vi "main.vi"() -> ()   [LabVIEW 2017]
panel:
  out "Resultado":dbl
  in  "Numero 2":dbl
  in  "Numero1":dbl
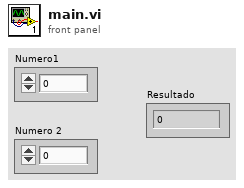
[diagram p1: front panel]
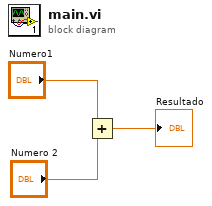
[diagram p0: block diagram]
diagram:
  n1 = Add(x="Numero1", y="Numero 2") -> (x+y=→"Resultado":dbl)
